vi "Drivetrain Encoder Read.vi"(6 "Reset?":bool) -> (2 "Quick use cluster":T1 {"Right Encoder"."Ticks" format="%#.6g"; "Center Encoder"."Ticks" format="%#.6g"; "Left Encoder"."Ticks" format="%#.6g"})   [LabVIEW 2014]
uses:
  Encoder Values SuperCluster.ctl
  Encoder Values.ctl
  Robot Global Data.vi
panel:
  in  "Encoder Values Super Cluster":T1 {"Right Encoder"."Ticks" format="%#.6g"; "Center Encoder"."Ticks" format="%#.6g"; "Left Encoder"."Ticks" format="%#.6g"}
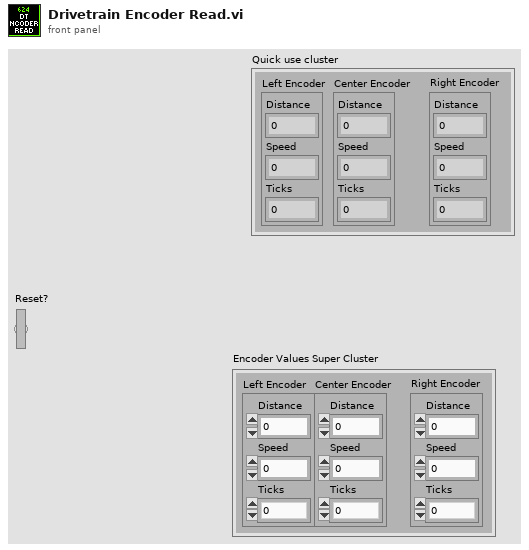
[diagram p1: front panel]
types:
  T1 = typedef "Encoder Values SuperCluster.ctl" = cluster{"Left Encoder":T2, "Center Encoder":T2, "Right Encoder":T2}
  T2 = typedef "Encoder Values.ctl" = cluster{"Distance":dbl, "Speed":dbl, "Ticks":dbl}
  T3 = typedef "Dashboard Control Data.ctl" = cluster{"Cam Exposure":dbl, "Go to angle":dbl, "Steer PID Gains":cluster{"proportional gain (Kc)":dbl, "integral time (Ti, min)":dbl, "derivative time (Td, min)":dbl}, "Steer PID output Range":cluster{"output high":dbl, "output low":dbl}, "Pressure m \nValue":dbl, "Pressure b \nValue":dbl, "Strafe Timer\nWait":dbl, "Roller Command Cluster ":T4, "Elevator":T5, "Strafe Correct min X":dbl, "IMU Enable":bool, "Encoder Control":T6}
  T4 = typedef "Roller Control.ctl" = cluster{"Left Roller Speed":dbl, "Right Roller Speed":dbl, "Left Roller Speed Back":dbl, "Right Roller Speed Back":dbl, "Roller Align Decide Limit":u32, "Left Roller Speed Unload":dbl, "Right Roller Speed Unload":dbl, "Ping Dist Difference":dbl}
  T5 = typedef "Elevator DB Control.ctl" = cluster{"PID Output Range":cluster{"output high":dbl, "output low":dbl}, "PID gains":cluster{"proportional gain (Kc)":dbl, "integral time (Ti, min)":dbl, "derivative time (Td, min)":dbl}, "Height Tolerance":dbl, " Encoder Constant":dbl, "Safe Mode Max Speed":dbl, "Presets":cluster{"Hold Tote":dbl, "Hold Trashcan":dbl, "Pickup 2 w/ Tote":dbl, "Pickup 2 w/ Trashcan":dbl, "Pickup 3 w/ Tote":dbl, "Pickup 3 w/ Trashcan":dbl, "Bottom":dbl, "Pickup 1 w/ Tote":dbl, "Pickup Trashcan":dbl, "Pickup 1 w/ Trashcan":dbl}}
  T6 = typedef "Encoder Control.ctl" = cluster{"Left Tick Constant":dbl, "Right Tick Constant":dbl, "Center Tick Constant":dbl, "Reset?":bool}
  T7 = typedef "WPI_EncoderDevRef.ctl" = cluster{"DevStatus":errorcluster, "EncoderIndex":T8, "CounterIndex":T9, "DistancePerCount":dbl, "Decoding Type":T10}
  T8 = typedef "FPGA_EncoderIdx.ctl" = enum8{"Enc 0", "Enc 1", "Enc 2", "Enc 3", "Enc 4", "Enc 5", "Enc 6", "Enc 7", "Invalid"}
  T9 = typedef "FPGA_CounterCtrSystemIndex.ctl" = enum8{"Ctr 0", "Ctr 1", "Ctr 2", "Ctr 3", "Ctr 4", "Ctr 5", "Ctr 6", "Ctr 7", "Invalid"}
  T10 = typedef "WPI_EncoderType.ctl" = enum16{"1x", "2x", "4x"}
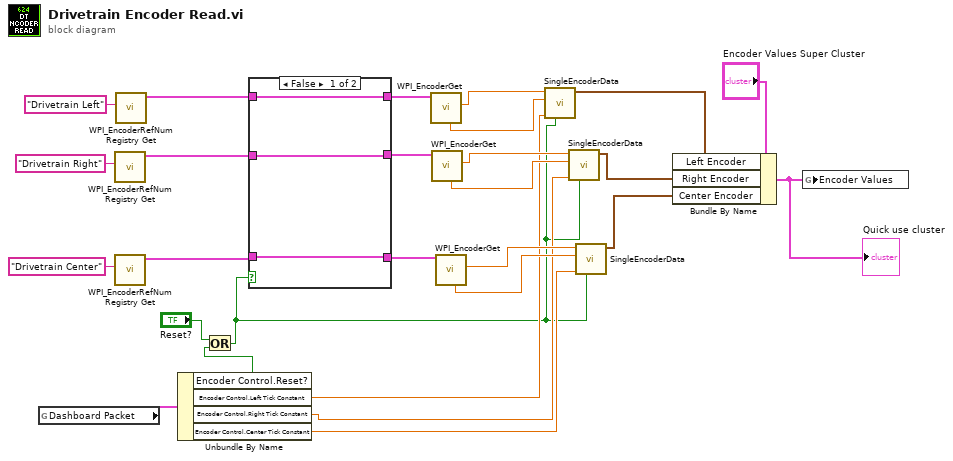
[diagram p0: block diagram]
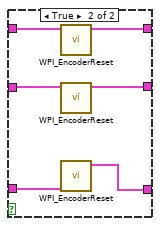
[diagram p2: hidden frame]
diagram:
  n1 = global read "Robot Global Data.vi" "Dashboard Packet"() -> (w7:T3)
  n2 = call <vilib>:"WPI_EncoderRefNum Registry Get.vi"("refnum name"="Drivetrain Right") -> ("EncoderDevRef"=w23:T7)  [unwired: 9 in, 1 out]
  n3 = call <vilib>:"WPI_EncoderRefNum Registry Get.vi"("refnum name"="Drivetrain Center") -> ("EncoderDevRef"=w24:T7)  [unwired: 9 in, 1 out]
  n4 = call <vilib>:"WPI_EncoderRefNum Registry Get.vi"("refnum name"="Drivetrain Left") -> ("EncoderDevRef"=w22:T7)  [unwired: 9 in, 1 out]
  n5 = Unbundle By Name(w7) -> ("Encoder Control.Reset?"=w1:bool, "Encoder Control.Left Tick Constant"=w6:dbl, "Encoder Control.Right Tick Constant"=w4:dbl, "Encoder Control.Center Tick Constant"=w5:dbl)
  n6 = Or(x="Reset?", y=w1) -> (x .or. y?=w2:bool)
  n7 = case shown="False" w2 {
    tunnel: w24 -> [w28 w35]
    tunnel: w23 -> [w29 w34]
    tunnel: w22 -> [w30 w36]
    tunnel: [w29 w33] -> w19
    tunnel: [w30 w32] -> w21
    tunnel: [w28 w31] -> w20
    frame False {
    }
    frame True {
      n8 = call <vilib>:"WPI_EncoderReset.vi"("EncoderDevRef"=w36) -> ("EncoderDevRef"=w32:T7)  [unwired: 9 in, 1 out]
      n9 = call <vilib>:"WPI_EncoderReset.vi"("EncoderDevRef"=w34) -> ("EncoderDevRef"=w33:T7)  [unwired: 9 in, 1 out]
      n10 = call <vilib>:"WPI_EncoderReset.vi"("EncoderDevRef"=w35) -> ("EncoderDevRef"=w31:T7)  [unwired: 9 in, 1 out]
    }
  }
  n11 = call <vilib>:"WPI_EncoderGet.vi"("EncoderDevRef"=w21) -> ("Distance"=w18:dbl, "Rate"=w17:dbl)  [unwired: 5 in, 4 out]
  n12 = call <vilib>:"WPI_EncoderGet.vi"("EncoderDevRef"=w19) -> ("Distance"=w16:dbl, "Rate"=w15:dbl)  [unwired: 5 in, 4 out]
  n13 = call <vilib>:"WPI_EncoderGet.vi"("EncoderDevRef"=w20) -> ("Distance"=w13:dbl, "Rate"=w14:dbl)  [unwired: 5 in, 4 out]
  n14 = call "SingleEncoderData.vi"("Reset?"=w2, "Tick Constant"=w6, "Rate"=w17, "Distance"=w18) -> ("Encoder Data"=w12:T2)  [unwired: 7 in]
  n15 = call "SingleEncoderData.vi"("Reset?"=w2, "Tick Constant"=w4, "Rate"=w15, "Distance"=w16) -> ("Encoder Data"=w11:T2)  [unwired: 7 in]
  n16 = call "SingleEncoderData.vi"("Reset?"=w2, "Tick Constant"=w5, "Rate"=w14, "Distance"=w13) -> ("Encoder Data"=w10:T2)  [unwired: 7 in]
  n17 = Bundle By Name(cluster="Encoder Values Super Cluster", "Left Encoder"=w12, "Right Encoder"=w11, "Center Encoder"=w10) -> (w8:T1)
  "Quick use cluster" <- w8
  n18 = global write "Robot Global Data.vi" "Encoder Values"(w8) -> ()
